vi "Shoot Mode - Drive Control Mode.vi"(0 "Post Speed Limit":dbl, 7 "Center of Mass X":dbl=300.8, 9 "reinitialize? (F)":bool=TRUE, 12 "Invert":bool=TRUE, 13 "PID gains":T1={"proportional gain (Kc)"=0.0036, "integral time (Ti, min)"=0.0, "derivative time (Td, min)"=0.008} {"derivative time (Td, min)" format="%.6f"; "integral time (Ti, min)" format="%.6f"; "proportional gain (Kc)" format="%.6f"}) -> ()   [LabVIEW 2012]
uses:
  <vilib>/addons/control/pid/pid.llb/PID (DBL).vi
  Globals/Robot Jaguars.vi
  <vilib>/addons/control/pid/NI_PID_pid.lvlib
panel:
  in  "Pre Speed Limit":cluster{"output high":dbl, "output low":dbl}={"output high"=1.0, "output low"=-1.0}
  out "output":dbl=0.06911999999999996 format="%.2f"
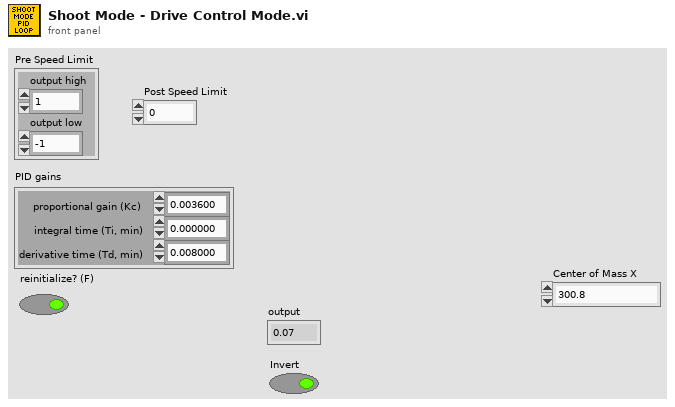
[diagram p1: front panel]
types:
  T1 = cluster{"proportional gain (Kc)":dbl, "integral time (Ti, min)":dbl, "derivative time (Td, min)":dbl}
  T2 = typedef "WPI_MotorControlDeviceRef.ctl" = cluster{"DeviceStatus":errorcluster, "Type":enum16{"PWM", "CAN"}, "PWM":cluster{"Digital Module":T3, "PWM Channel":T4, "DeadBand":T5}, "CAN":cluster{"Device Number":u8, "Control Mode":T6, "Semaphore":T7, "Max Vout":dbl}, "Invert":bool, "TransformRef":T8, "InvTransformRef":T8}
  T3 = typedef "FPGA_TypedefDigitalModule.ctl" = enum16{"Digital Module 1", "Digital Module 2"}
  T4 = typedef "FPGA_DIOPWMChannel.ctl" = enum8{"PWM 1", "PWM 2", "PWM 3", "PWM 4", "PWM 5", "PWM 6", "PWM 7", "PWM 8", "PWM 9", "PWM 10", "Invalid"}
  T5 = typedef "WPI_PWMDeadband.ctl" = cluster{"Name":string, "maxPositivePwm":i32, "minPositivePwm":i32, "centerPwm":i32, "maxNegativePwm":i32, "minNegativePwm":i32, "angularRange":u16}
  T6 = typedef "WPI_CANJaguar_ControlMode.ctl" = enum8{"Percent VBus", "Current", "Speed", "Position", "Voltage"}
  T7 = typedef "Semaphore RefNum" = refnum<k1>
  T8 = typedef "WPI_PWMTransform_ConPane.ctl" = refnum<vi>
  T9 = cluster{"Front Left Drive":T2, "Front Right Drive":T2, "Rear Left Drive":T2, "Rear Right Drive":T2, "Front Left Steer":T2, "Front Right Steer":T2, "Rear Left Steer":T2, "Rear Right Steer":T2}
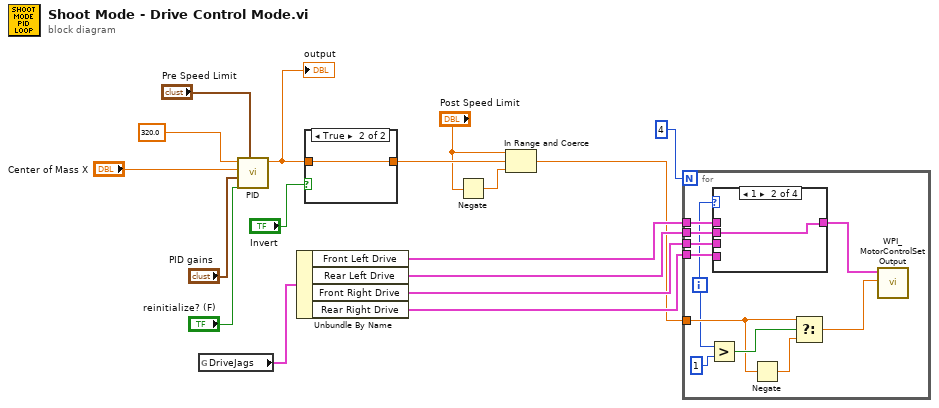
[diagram p0: block diagram]
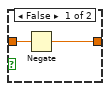
[diagram p5: hidden frame]
diagram:
  n1 = global read "Robot Jaguars.vi" "DriveJags"() -> (w12:T9)
  n2 = call-poly <vilib>:"PID.vi"("reinitialize? (F)"="reinitialize? (F)", "output range"="Pre Speed Limit", "PID gains"="PID gains", "process variable"="Center of Mass X", "setpoint"=320.0) -> ("output"=w14:dbl)  [unwired: 5 in, 1 out]
  "output" <- w14
  n3 = Unbundle By Name(w12) -> ("Front Left Drive"=w11:T2, "Rear Left Drive"=w10:T2, "Front Right Drive"=w9:T2, "Rear Right Drive"=w8:T2)
  n4 = case shown="True" "Invert" {
    tunnel: w14 -> [w19 w20]
    tunnel: [w18 w20] -> w7
    frame False {
      n5 = Negate(x=w19) -> (-x=w18:dbl)
    }
    frame True {
    }
  }
  n6 = Negate(x="Post Speed Limit") -> (-x=w2:dbl)
  n7 = In Range and Coerce(upper limit="Post Speed Limit", x=w7, lower limit=w2) -> (coerced(x)=w3:dbl)  [unwired: 1 out]
  n8 = for {
    N: 4 -> [_]
    tunnel: w11 -> [w31]
    tunnel: w10 -> [w30]
    tunnel: w9 -> [w29]
    tunnel: w8 -> [w28]
    tunnel: w3 -> [w24]
    i -> [w23]
    n9 = Greater?(x=w23, y=1) -> (0:w26:bool)
    n10 = case shown="1" w23 {
      tunnel: w31 -> [w32 _ _ _]
      tunnel: w30 -> [_ w33 _ _]
      tunnel: w29 -> [_ _ w34 _]
      tunnel: w28 -> [_ _ _ w35]
      tunnel: [w32 w33 w34 w35] -> w27
      frame 0, Default {
      }
      frame 1 {
      }
      frame 2 {
      }
      frame 3 {
      }
    }
    n11 = Negate(x=w24) -> (-x=w25:dbl)
    n12 = Select(t=w24, s=w26, f=w25) -> (s? t:f=w21:dbl)
    n13 = call <vilib>:"WPI_MotorControlSetOutput.vi"("Output"=w21, "MotorControlDevRef"=w27) -> ()  [unwired: 7 in, 3 out]
  }
